vi "Launch Thread.vi"(8 "error in (no error)":errorcluster, 11 "WebSocket in":refnum<class "WebSocket.lvclass">) -> (0 "error out":errorcluster, 3 "WebSocket out":refnum<class "WebSocket.lvclass">)   [LabVIEW 2023, in "WebSocket.lvclass"]
uses:
  WebSocket.lvclass
  Log/Log_Facilities.ctl
  Log/Log.lvclass
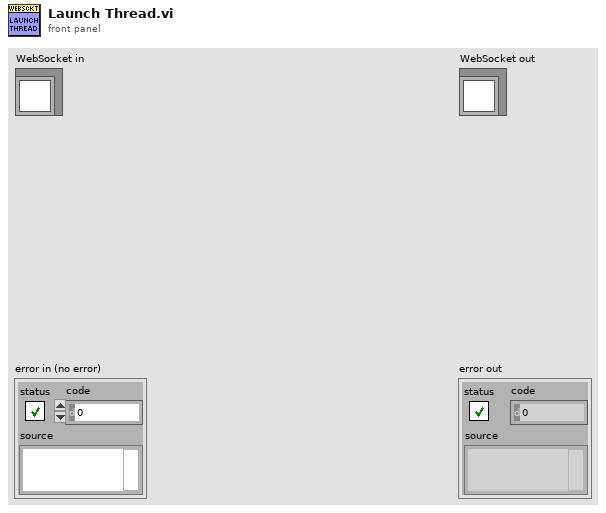
[diagram p1: front panel]
types:
  T1 = typedef "Log.lvclass/Log_Facilities.ctl" = string
  T2 = typedef "WebSocket.lvclass/ObjectAttributes.ctl" = cluster{"Socket":refnum<k5>, "Thread":refnum<vi>, "From Socket":refnum<queue>, "To Socket":refnum<queue>, "Rx Stats in Progress":variant, "Rx Stats":variant, "Tx Stats in Progress":variant, "Tx Stats":variant}
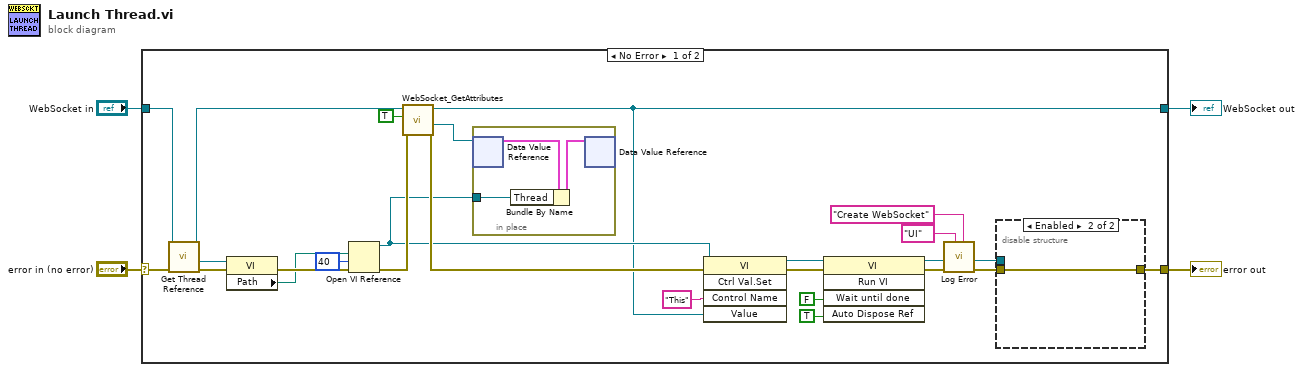
[diagram p0: block diagram]
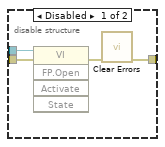
[diagram p2: hidden frame]
diagram:
  n1 = case shown="No Error" "error in (no error)" {
    selector: "error in (no error)" -> [w20 w39]
    tunnel: [w8 w39] -> w3
    tunnel: [w9 w38] -> w1
    tunnel: "WebSocket in" -> [w21 w38]
    frame No Error {
      n2 = call-dynamic "Get Thread Reference.vi"("error in (no error)"=w20, "WebSocket in"=w21) -> ("error out"=w19:errorcluster, "Thread VI"=w18:refnum<vi>, "WebSocket out"=w14:refnum<class "WebSocket.lvclass">)  [unwired: 7 in]
      n3 = property class="VI"(reference=w18, error in=w19) -> (error out=w29:errorcluster, "Path"=w28:path)  [unwired: 1 out]
      n4 = Open VI Reference(vi path=w28, options=40, error in (no error)=w29) -> (vi reference=w10:refnum<vi>, error out=w13:errorcluster)  [unwired: 3 in]
      n5 = call "WebSocket_GetAttributes.vi"("error in (no error)"=w13, "OnlyGetDvrReference(False)"=TRUE, "reference in"=w14) -> ("error out"=w12:errorcluster, "DataRef"=w15:refnum<data-value>, "reference out"=w9:refnum<class "WebSocket.lvclass">)  [unwired: 5 in, 1 out]
      n6 = in-place {
        in-place-border: w10 -> [w30]
        n7 = in-place-dvr #1(w15) -> (w32:T2)  [unwired: 1 out]
        n8 = Bundle By Name(cluster=w32, "Thread"=w30) -> (w31:T2)
        n9 = in-place-dvr #1(w31) -> ()  [unwired: 2 out]
      }
      n10 = invoke class="VI" method="Ctrl Val.Set"(reference=w10, error in=w12, "Control Name"="This", "Value"=w9) -> (reference out=w24:refnum<vi>, error out=w26:errorcluster)  [unwired: 1 in, 3 out]
      n11 = invoke class="VI" method="Run VI"(reference=w24, error in=w26, "Wait until done"=FALSE ("Wait Until Done"), "Auto Dispose Ref"=TRUE ("Auto Dispose Reference")) -> (reference out=w17:refnum<vi>, error out=w16:errorcluster)  [unwired: 1 in, 3 out]
      n12 = call "Log Error.vi"("Context"="Create WebSocket" ("Control Name"), "Facility (default)"=T1 "UI", "error in (no error)"=w16) -> ("error out"=w7:errorcluster)  [unwired: 8 in]
      n13 = disable-structure shown="Enabled" {
        disable-tunnel: w17 -> [w36 _]
        disable-tunnel: w7 -> [w35 w37]
        disable-tunnel: [w33 w37] -> w8
        frame Disabled {
          n14 = invoke class="VI" method="FP.Open"(reference=w36, error in=w35) -> (error out=w34:errorcluster)  [unwired: 3 in, 4 out]
          n15 = call <vilib>:"Clear Errors.vi"("error in (no error)"=w34) -> ("error out"=w33:errorcluster)  [unwired: 5 in, 1 out]
        }
        frame Enabled {
        }
      }
    }
    frame Error {
    }
  }
  "error out" <- w3
  "WebSocket out" <- w1
